vi "ALU.vi"(4 "S - 1":bool, 5 "5":bool, 6 "?":bool, 7 "?":bool, 8 "4":bool, 9 "3":bool, 10 "2":bool, 11 "1":bool) -> (0 "cf":bool, 2 "S":bool)   [LabVIEW 2017]
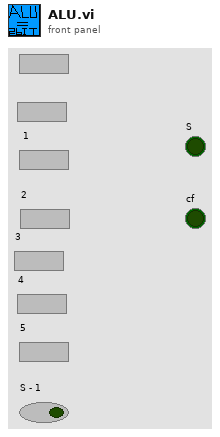
[diagram p1: front panel]
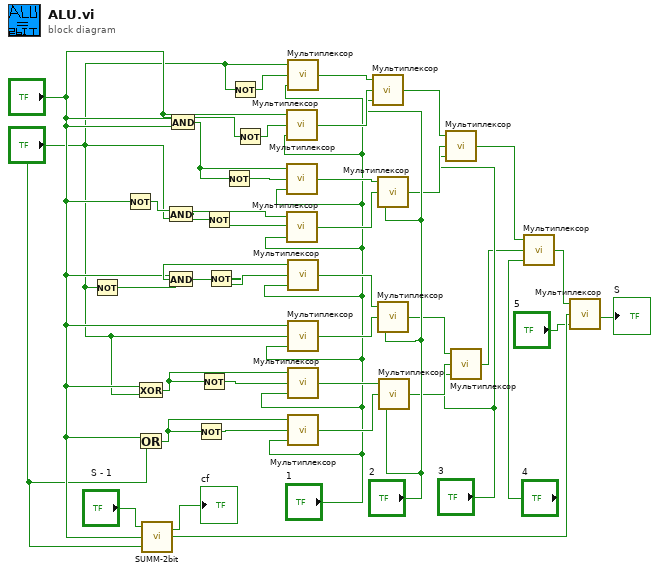
[diagram p0: block diagram]
diagram:
  n1 = Not(x="?") -> (.not. x?=w39:bool)
  n2 = Not(x="?") -> (.not. x?=w40:bool)
  n3 = Exclusive Or(1:"?", 2:"?") -> (0:w33:bool)
  n4 = Or(x="?", y="?") -> (x .or. y?=w31:bool)
  n5 = call "SUMM-2bit.vi"("b0"="?", "a0"="?", "OP"="S - 1") -> ("S0"=w6:bool, "S1"=→"cf":bool)
  n6 = And(x=w40, y="?") -> (x .and. y?=w27:bool)
  n7 = And(x="?", y=w39) -> (x .and. y?=w34:bool)
  n8 = And(x="?", y="?") -> (x .and. y?=w29:bool)
  n9 = Not(x=w31) -> (.not. x?=w30:bool)
  n10 = Not(x=w33) -> (.not. x?=w32:bool)
  n11 = Not(x=w27) -> (.not. x?=w36:bool)
  n12 = Not(x=w34) -> (.not. x?=w35:bool)
  n13 = Not(x=w29) -> (.not. x?=w28:bool)
  n14 = Not(x="?") -> (.not. x?=w38:bool)
  n15 = Not(x="?") -> (.not. x?=w37:bool)
  n16 = call "Мультиплексор.vi"(1:"1", "2"=w37, "1"="?") -> (0:w20:bool)
  n17 = call "Мультиплексор.vi"(1:"1", "2"=w28, "1"=w29) -> (0:w21:bool)
  n18 = call "Мультиплексор.vi"(1:"1", "2"=w36, "1"=w27) -> (0:w22:bool)
  n19 = call "Мультиплексор.vi"(1:"1", "2"=w38, "1"="?") -> (0:w19:bool)
  n20 = call "Мультиплексор.vi"(1:"1", "2"=w35, "1"=w34) -> (0:w23:bool)
  n21 = call "Мультиплексор.vi"(1:"1", "2"="?", "1"="?") -> (0:w24:bool)
  n22 = call "Мультиплексор.vi"(1:"1", "2"=w32, "1"=w33) -> (0:w25:bool)
  n23 = call "Мультиплексор.vi"(1:"1", "2"=w30, "1"=w31) -> (0:w26:bool)
  n24 = call "Мультиплексор.vi"(1:"2", "2"=w20, "1"=w19) -> (0:w14:bool)
  n25 = call "Мультиплексор.vi"(1:"2", "2"=w22, "1"=w21) -> (0:w15:bool)
  n26 = call "Мультиплексор.vi"(1:"2", "2"=w24, "1"=w23) -> (0:w16:bool)
  n27 = call "Мультиплексор.vi"(1:"2", "2"=w26, "1"=w25) -> (0:w17:bool)
  n28 = call "Мультиплексор.vi"(1:"3", "2"=w15, "1"=w14) -> (0:w10:bool)
  n29 = call "Мультиплексор.vi"(1:"3", "2"=w17, "1"=w16) -> (0:w11:bool)
  n30 = call "Мультиплексор.vi"(1:"4", "2"=w11, "1"=w10) -> (0:w7:bool)
  n31 = call "Мультиплексор.vi"(1:"5", "2"=w6, "1"=w7) -> (0:→"S":bool)
